vi "test motor reactions.vi"(6 "testing?":bool, 8 "REF INPUT":cluster{T30[], T36[], T39[], T40[], T41[]}={[{"Device"=enum."USB 0"}], [{"DevStatus"={"status"=FALSE, "code"=0, "source"=""}, "EncoderIndex"=enum."Enc 0", "CounterIndex"=enum."Invalid", "DistancePerCount"=0.026179938779914938, "Decoding Type"=enum."4x"}, {"DevStatus"={"status"=FALSE, "code"=0, "source"=""}, "EncoderIndex"=enum."Enc 1", "CounterIndex"=enum."Invalid", "DistancePerCount"=0.026179938779914938, "Decoding Type"=enum."4x"}], [], [], []}, 9 "REF OUTPUT":cluster{T32[], T42[], T43[]}, 10 "HARDWARE cluster":T1={"DRIVE MOTORS"=[], "Controller"=[], "ENCODERS"=[], "GYRO HARDWARE"={"Descr"="GYRO", "Installed?"=FALSE, "SPI Bus"=enum."SPI On-Board, CS0", "AnalogChannel"=enum."AI 0", "Calibrate On Open"=TRUE, "Calibrated Center Voltage"=0.0, "Calibration Time (s)"=2.0, "Sample Rate (Hz)"=100.0, "RefName"="", "stack name"="GYRO"}, "AIR"={"PRESSURE"=[], "COMPRESSOR"={"Descr"="COMPRESSOR", "Installed?"=TRUE, "Pneumatics Control Module"=0, "RefName"="COMPRESSOR", "stack name"="COMPRESSOR"}, "SOLENOIDS"=[]}, "MOTORS"=[], "SERVOS"=[], "SONAR"=[], "RELAY"=[], "LIMIT"=[]} {"MOTORS"."CAN ID" min=1 max=62 step=1; "MOTORS"."Motor Controller" items=["SPARK MAX", "SPARK", "Existing", "SD540", "TALON SRX", "VICTOR SP", "TALON SR", "JAGUAR", "VICTOR"]; "AIR"."PRESSURE"."warning HIGH" format="%.2f"; "AIR"."PRESSURE"."warning LOW" format="%.2f"; "AIR"."PRESSURE"."nominal value" format="%.2f"; "DRIVE MOTORS"."CAN ID" min=1 max=62 step=1; "DRIVE MOTORS"."Motor Controller" items=["SPARK MAX", "SPARK", "Existing", "SD540", "TALON SRX", "VICTOR SP", "TALON SR", "JAGUAR", "VICTOR"]; "Controller"."Parameters"."DEADBAND" format="%#_13g"; "Controller"."Parameters"."MIN SPEED" format="%#_13g"; "Controller"."Parameters"."MAX LIMIT" format="%#_13g"}, 11 "REF DRIVE JOYSTICK":T35={"JoystickDevRef"={"Device"=enum."USB 0"}, "RobotDriveDevRef"={"DevStatus"={"status"=FALSE, "code"=0, "source"=""}, "Motors[]"=[{"DeviceStatus"={"status"=FALSE, "code"=0, "source"=""}, "Type"=enum."PWM", "PWM"={"PWM Channel"=enum."PWM 0", "DeadBand"={"Name"="Victor SP", "maxPositivePwm"=230, "minPositivePwm"=154, "centerPwm"=153, "maxNegativePwm"=152, "minNegativePwm"=76, "angularRange"=0}}, "CAN"={"Device Number"=0, "SetOutput VI Ref"=variant(enum8{"Percent VBus", "Current", "Speed", "Position", "Voltage"} enum."Percent VBus"), "GetOutput VI Ref"=variant(refnum<k1> refnum), "Enable VI Ref"=variant(dbl 0.0), "Disable VI Ref"=variant(enum8{"Percent VBus", "Speed", "Position", "Slave", "Unchanged / Invalid"} enum."Percent VBus"), "Data"=variant}, "Invert"=FALSE, "DIO PWM"={"PWM \"Enable\" Channel"=enum."Invalid", "DIOChannel"=enum."Invalid", "PWM Rate"=0.0}}, {"DeviceStatus"={"status"=FALSE, "code"=0, "source"=""}, "Type"=enum."PWM", "PWM"={"PWM Channel"=enum."PWM 1", "DeadBand"={"Name"="Victor SP", "maxPositivePwm"=230, "minPositivePwm"=154, "centerPwm"=153, "maxNegativePwm"=152, "minNegativePwm"=76, "angularRange"=0}}, "CAN"={"Device Number"=0, "SetOutput VI Ref"=variant(enum8{"Percent VBus", "Current", "Speed", "Position", "Voltage"} enum."Percent VBus"), "GetOutput VI Ref"=variant(refnum<k1> refnum), "Enable VI Ref"=variant(dbl 0.0), "Disable VI Ref"=variant(enum8{"Percent VBus", "Speed", "Position", "Slave", "Unchanged / Invalid"} enum."Percent VBus"), "Data"=variant}, "Invert"=TRUE, "DIO PWM"={"PWM \"Enable\" Channel"=enum."Invalid", "DIOChannel"=enum."Invalid", "PWM Rate"=0.0}}], "Square Inputs"=TRUE, "Max Output"=1.0}}) -> (2 "Cluster":cluster{"LEFT":dbl, "RIGHT":dbl}={"LEFT"=155.04062951459707, "RIGHT"=154.7082225850084})   [LabVIEW 2019]
uses:
  <vilib>/Rock Robotics/WPI/MotorControl/WPI_MotorControlDeviceRef.ctl
  <vilib>/Rock Robotics/WPI/MotorControl/WPI_MotorControlType.ctl
  <vilib>/Rock Robotics/SystemInterfaces/DIO/FPGA_DIOPWMChannel.ctl
  <vilib>/Rock Robotics/WPI/PWM/WPI_PWMDeadband.ctl
  <vilib>/Rock Robotics/SystemInterfaces/DIO/FPGA_DIOChannel.ctl
  <vilib>/Rock Robotics/WPI/PWM/Servo/WPI_ServoDeviceRef.ctl
  <vilib>/Rock Robotics/WPI/Relay/WPI_RelayDevRef.ctl
  <vilib>/Rock Robotics/SystemInterfaces/DIO/FPGA_DIORelayChannel.ctl
  <vilib>/Rock Robotics/WPI/Relay/WPI_RelayDirection.ctl
  <vilib>/Rock Robotics/WPI/Joystick/WPI_JoystickDevRef.ctl
  <vilib>/Rock Robotics/WPI/Joystick/WPI_JoystickDeviceEnum.ctl
  <vilib>/Rock Robotics/WPI/Encoder/WPI_EncoderDevRef.ctl
  <vilib>/Rock Robotics/SystemInterfaces/Encoder/FPGA_EncoderIdx.ctl
  <vilib>/Rock Robotics/SystemInterfaces/Counter/FPGA_CounterCtrSystemIndex.ctl
  <vilib>/Rock Robotics/WPI/Encoder/WPI_EncoderType.ctl
  <vilib>/Rock Robotics/WPI/Ultrasonic/WPI_UltrasonicDeviceRef.ctl
  <vilib>/Rock Robotics/WPI/Switch/WPI_SwitchDevRef.ctl
  <vilib>/Rock Robotics/WPI/AnalogChannel/WPI_AnalogChannelDevRef.ctl
  <vilib>/Rock Robotics/SystemInterfaces/AI/FPGA_AIChannel.ctl
  <vilib>/Rock Robotics/WPI/RobotDrive/WPI_RobotDriveDevRef.ctl
  Controls/def HARDWARE CTRL info.ctl
  Controls/def MOTOR info.ctl
  Controls/ctrl MOTOR CTRLR SELECT.ctl
  <vilib>/Rock Robotics/WPI/ThirdParty/REV Robotics/SPARK MAX/Typedef/Spark MAX Motor Type.ctl
  Controls/def USER CONTROL info.ctl
  Controls/def JOYSTICK PARAMETERS.ctl
  Controls/def ENCODER info.ctl
  Controls/def GYRO info.ctl
  <vilib>/Rock Robotics/SystemInterfaces/spilib/spi_bus.ctl
  Controls/ctrl ANALOG CHANNEL SELECT.ctl
  Controls/def AIR PRESSURE info.ctl
  Controls/def COMPRESSOR info.ctl
  Controls/def SOLENOID info.ctl
  <vilib>/Rock Robotics/WPI/Solenoid/WPI_SolenoidChannel.ctl
  <vilib>/Rock Robotics/WPI/Solenoid/WPI_SolenoidValue.ctl
  Controls/def SERVO info.ctl
  Controls/def SONAR info.ctl
  Controls/ctrl SONAR DEVICE SELECT.ctl
  <vilib>/Rock Robotics/WPI/Ultrasonic/WPI_UltrasonicRangeUnits.ctl
  Controls/def RELAY info.ctl
  <vilib>/Rock Robotics/WPI/Relay/WPI_RelayValue.ctl
  Controls/def LIMIT SWITCH info.ctl
  Controls/ctrl ENCODER SELECT.ctl
panel:
  in  "milliseconds to wait":u32=25
  in  "INNER LOOPS":i32=50
  out "v":cluster{"LEFT":dbl, "RIGHT":dbl}={"LEFT"=34.73439216613769, "RIGHT"=34.65523719787597}
  out "x":cluster{"LEFT":dbl, "RIGHT":dbl}={"LEFT"=155.04062951459707, "RIGHT"=154.7082225850084}
  out "size(s)":i32=2
  out "Waveform Chart":T44(graph)=[{11.395975494291633, "Numeric"=1.0, "LEFT"=155.04062951459707, "RIGHT"=154.7082225850084, "LEFT"=34.73439216613769, "RIGHT"=34.65523719787597}]
  out "elapsed t (s)":dbl=11.395975494291633 format="%.4f"
  out "delta t (s)":dbl=0.05002135713584721 format="%.4f"
  out "MOTOR VALUE":dbl=1.0
  out "motor profile":dbl[](array[numeric])=[0.0, 0.05, 0.1, 0.15000000000000002, 0.2, 0.25, 0.30000000000000004, 0.35000000000000003, 0.4, 0.45, 0.5, 0.55, 0.6000000000000001, 0.65, 0.7000000000000001, 0.75, 0.8, 0.8500000000000001, 0.9, 0.9500000000000001, 1.0] format="%.3f"
  in  "motor increment":dbl=0.05 format="%#_13g"
  in  "motor profile type":enum16{"unit pulse", "step"}(ring)
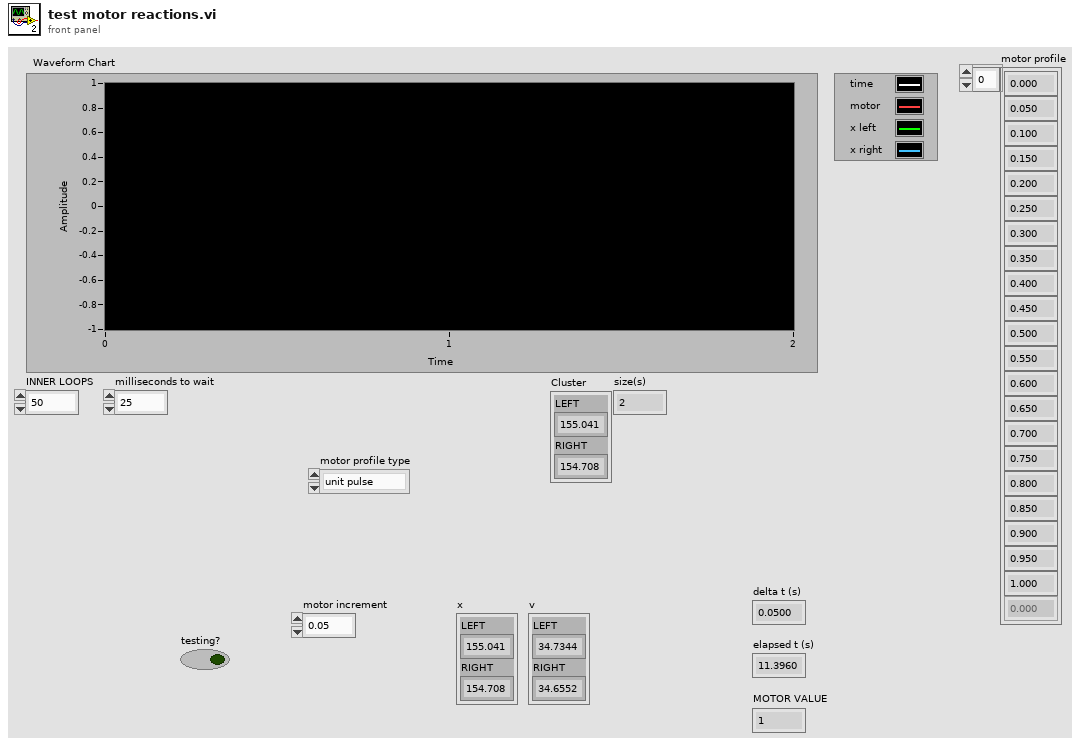
[diagram p1: front panel]
types:
  T1 = typedef "def HARDWARE CTRL info.ctl" = cluster{"DRIVE MOTORS":T2[], "Controller":T6[], "ENCODERS":T9[], "GYRO HARDWARE":T12, "AIR":cluster{"PRESSURE":T15[], "COMPRESSOR":T17, "SOLENOIDS":T18[]}, "MOTORS":T2[], "SERVOS":T21[], "SONAR":T22[], "RELAY":T25[], "LIMIT":T29[]}
  T2 = typedef "def MOTOR info.ctl" = cluster{"Descr":string, "Motor Controller":T3, "PWM ch":T4, "Invert?":bool, "Installed?":bool, "RefName":string, "stack name":string, "remove deadband":bool, "CAN ID":u8, "IDLE BEHAVIOUR":string, "Motor Type":T5}
  T3 = typedef "ctrl MOTOR CTRLR SELECT.ctl" = u16
  T4 = typedef "FPGA_DIOPWMChannel.ctl" = enum8{"PWM 0", "PWM 1", "PWM 2", "PWM 3", "PWM 4", "PWM 5", "PWM 6", "PWM 7", "PWM 8", "PWM 9", "PWM MXP 0", "PWM MXP 1", "PWM MXP 2", "PWM MXP 3", "PWM MXP 4", "PWM MXP 5", "PWM MXP 6", "PWM MXP 7", "PWM MXP 8", "PWM MXP 9", "Invalid"}
  T5 = typedef "Spark MAX Motor Type.ctl" = enum16{"Brushed", "Brushless"}
  T6 = typedef "def USER CONTROL info.ctl" = cluster{"Descr":string, "Installed?":bool, "RefName":string, "JoystickDevice":T7, "Invert Y axis":bool, "Scale":dbl, "AXIS":string, "BUTTONS":string, "POV":string, "Parameters":T8}
  T7 = typedef "WPI_JoystickDeviceEnum.ctl" = enum16{"USB 0", "USB 1", "USB 2", "USB 3", "USB 4", "USB 5"}
  T8 = typedef "def JOYSTICK PARAMETERS.ctl" = cluster{"MAX LIMIT":dbl, "MIN SPEED":dbl, "DEADBAND":dbl, "invert X?":bool, "invert Y?":bool}
  T9 = typedef "def ENCODER info.ctl" = cluster{"Descr":string, "Installed?":bool, "A Channel":T10, "B Channel":T10, "Invert Direction":bool, "Enum":T11, "Gear ratio":dbl, "Cycles per Rev":dbl, "Diameter (in)":dbl[unit], "RefName":string, "stack name":string, "min rate (hz)":dbl, "Samples":u8, "STACK subnames":cluster{"RESET name":string, "STOPPED name":string, "DIRECTION name":string, "RATE name":string, "INSTALLED name":string}}
  T10 = typedef "FPGA_DIOChannel.ctl" = enum8{"DIO 0", "DIO 1", "DIO 2", "DIO 3", "DIO 4", "DIO 5", "DIO 6", "DIO 7", "DIO 8", "DIO 9", "DIO MXP 0", "DIO MXP 1", "DIO MXP 2", "DIO MXP 3", "DIO MXP 4", "DIO MXP 5", "DIO MXP 6", "DIO MXP 7", "DIO MXP 8", "DIO MXP 9", "DIO MXP 10", "DIO MXP 11", "DIO MXP 12", "DIO MXP 13", "DIO MXP 14", "DIO MXP 15", "SPI Port CS1", "SPI Port CS2", "SPI Port CS3", "SPI Port MISO", "SPI Port MOSI", "Invalid"}
  T11 = typedef "WPI_EncoderType.ctl" = enum16{"1x", "2x", "4x"}
  T12 = typedef "def GYRO info.ctl" = cluster{"Descr":string, "Installed?":bool, "SPI Bus":T13, "AnalogChannel":T14, "Calibrate On Open":bool, "Calibrated Center Voltage":dbl, "Calibration Time (s)":dbl, "Sample Rate (Hz)":dbl, "RefName":string, "stack name":string}
  T13 = typedef "spi_bus.ctl" = enum16{"SPI On-Board, CS0", "SPI On-Board, CS1", "SPI On-Board, CS2", "SPI On-Board, CS3", "SPI MXP", "Invalid"}
  T14 = typedef "ctrl ANALOG CHANNEL SELECT.ctl" = enum8{"AI 0", "AI 1", "Invalid"}
  T15 = typedef "def AIR PRESSURE info.ctl" = cluster{"Descr":string, "Installed?":bool, "Channel":T16, "RefName":string, "stack name":string, "MULTIPLIER":dbl, "OFFSET":dbl, "nominal value":dbl, "warning LOW":dbl, "warning HIGH":dbl}
  T16 = typedef "FPGA_AIChannel.ctl" = enum8{"AI 0", "AI 1", "AI 2", "AI 3", "AI MXP 0", "AI MXP 1", "AI MXP 2", "AI MXP 3", "Invalid"}
  T17 = typedef "def COMPRESSOR info.ctl" = cluster{"Descr":string, "Installed?":bool, "Pneumatics Control Module":u8, "RefName":string, "stack name":string}
  T18 = typedef "def SOLENOID info.ctl" = cluster{"Descr":string, "Installed?":bool, "Pneumatics Control Module (0)":u8, "DBL":bool, "SolenoidChannel":T19, "SolenoidChannel":T19, "Default SET":T20, "RefName":string, "Value":string}
  T19 = typedef "WPI_SolenoidChannel.ctl" = enum8{"Solenoid 0", "Solenoid 1", "Solenoid 2", "Solenoid 3", "Solenoid 4", "Solenoid 5", "Solenoid 6", "Solenoid 7", "Invalid"}
  T20 = typedef "WPI_SolenoidValue.ctl" = enum16{"Off", "On", "Forward", "Reverse"}
  T21 = typedef "def SERVO info.ctl" = cluster{"Descr":string, "PWM ch":T4, "Installed?":bool, "Angular range":dbl, "RefName":string, "stack name":string}
  T22 = typedef "def SONAR info.ctl" = cluster{"Descr":string, "Installed?":bool, "Device type":T23, "PING Channel":T10, "ECHO Channel":T10, "RefName":string, "stack name":string, "Samples":i32, "Range Units":T24}
  T23 = typedef "ctrl SONAR DEVICE SELECT.ctl" = enum16{"SRF04 Digital", "MB1010 Digital", "MB1010 Analog", "SRF08 Digital"}
  T24 = typedef "WPI_UltrasonicRangeUnits.ctl" = enum16{"inches", "mm"}
  T25 = typedef "def RELAY info.ctl" = cluster{"Descr":string, "Installed?":bool, "RelayChannel":T26, "Relay Direction":T27, "Relay Value":T28, "RefName":string, "Value":string}
  T26 = typedef "FPGA_DIORelayChannel.ctl" = enum8{"Relay 0", "Relay 1", "Relay 2", "Relay 3", "Invalid"}
  T27 = typedef "WPI_RelayDirection.ctl" = enum16{"Both directions", "Forward only", "Reverse only"}
  T28 = typedef "WPI_RelayValue.ctl" = enum16{"Off", "On", "Forward", "Reverse"}
  T29 = typedef "def LIMIT SWITCH info.ctl" = cluster{"Descr":string, "Installed?":bool, "A Channel":T10, "Normally Closed?":bool, "RefName":string, "stack name":string}
  T30 = typedef "WPI_JoystickDevRef.ctl" = cluster{"Device":T7}
  T31 = typedef "WPI_RobotDriveDevRef.ctl" = cluster{"DevStatus":errorcluster, "Motors[]":T32[], "Square Inputs":bool, "Max Output":dbl}
  T32 = typedef "WPI_MotorControlDeviceRef.ctl" = cluster{"DeviceStatus":errorcluster, "Type":T33, "PWM":cluster{"PWM Channel":T4, "DeadBand":T34}, "CAN":cluster{"Device Number":u8, "SetOutput VI Ref":variant, "GetOutput VI Ref":variant, "Enable VI Ref":variant, "Disable VI Ref":variant, "Data":variant}, "Invert":bool, "DIO PWM":cluster{"PWM \"Enable\" Channel":T4, "DIOChannel":T10, "PWM Rate":dbl}}
  T33 = typedef "WPI_MotorControlType.ctl" = enum16{"PWM", "CAN", "DIO PWM"}
  T34 = typedef "WPI_PWMDeadband.ctl" = cluster{"Name":string, "maxPositivePwm":i32, "minPositivePwm":i32, "centerPwm":i32, "maxNegativePwm":i32, "minNegativePwm":i32, "angularRange":u16}
  T35 = cluster{"JoystickDevRef":T30, "RobotDriveDevRef":T31}
  T36 = typedef "WPI_EncoderDevRef.ctl" = cluster{"DevStatus":errorcluster, "EncoderIndex":T37, "CounterIndex":T38, "DistancePerCount":dbl, "Decoding Type":T11}
  T37 = typedef "FPGA_EncoderIdx.ctl" = enum8{"Enc 0", "Enc 1", "Enc 2", "Enc 3", "Enc 4", "Enc 5", "Enc 6", "Enc 7", "Invalid"}
  T38 = typedef "FPGA_CounterCtrSystemIndex.ctl" = enum8{"Ctr 0", "Ctr 1", "Ctr 2", "Ctr 3", "Ctr 4", "Ctr 5", "Ctr 6", "Ctr 7", "Invalid"}
  T39 = typedef "WPI_UltrasonicDeviceRef.ctl" = cluster{"DevStatus":errorcluster, "Ping Channel":T10, "Echo Channel":T10, "CntIndex":T38}
  T40 = typedef "WPI_SwitchDevRef.ctl" = cluster{"DevStatus":errorcluster, "DIO Channel":T10, "CntIndex":T38, "Normally Closed":bool}
  T41 = typedef "WPI_AnalogChannelDevRef.ctl" = cluster{"DevStatus":errorcluster, "Analog Channel":T16}
  T42 = typedef "WPI_ServoDeviceRef.ctl" = cluster{"DeviceStatus":errorcluster, "PWM Channel":T4, "DeadBand":T34}
  T43 = typedef "WPI_RelayDevRef.ctl" = cluster{"DevStatus":errorcluster, "Relay Channel":T26, "Relay Direction":T27}
  T44 = cluster{dbl, "Numeric":dbl, "LEFT":dbl, "RIGHT":dbl, "LEFT":dbl, "RIGHT":dbl}[]
  T45 = cluster{dbl, "Numeric":dbl, "LEFT":dbl, "RIGHT":dbl, "LEFT":dbl, "RIGHT":dbl}
  T46 = typedef "ctrl ENCODER SELECT.ctl" = u16
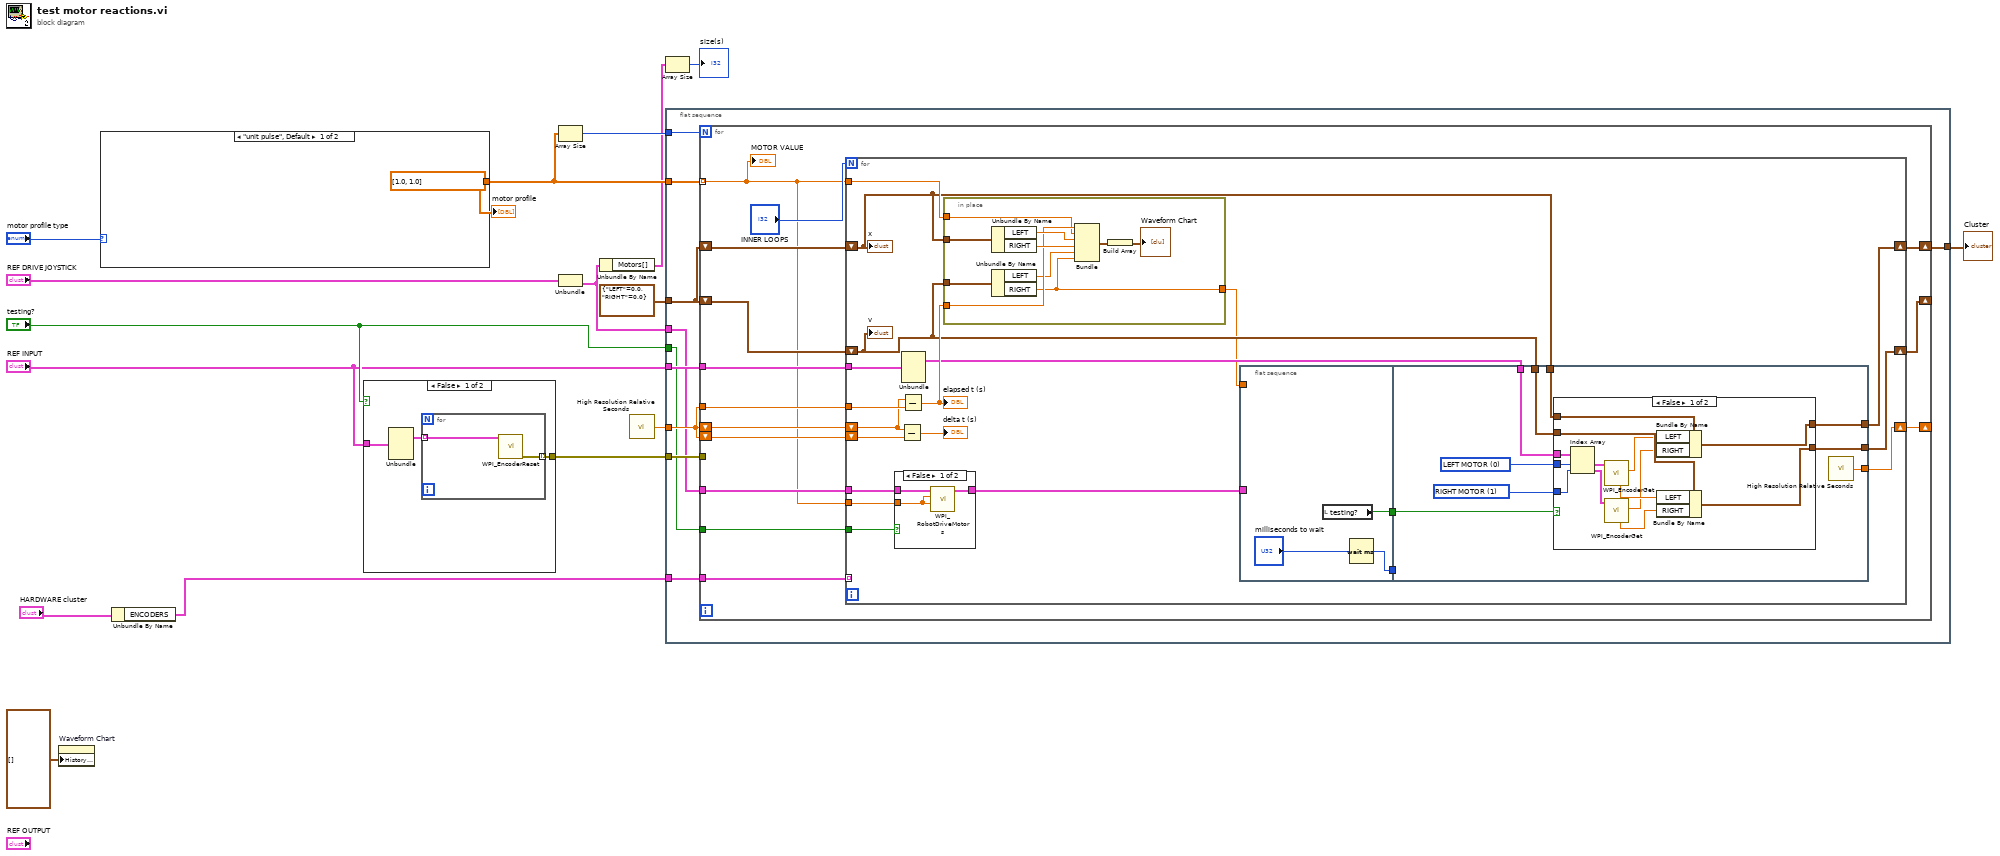
[diagram p0: block diagram]
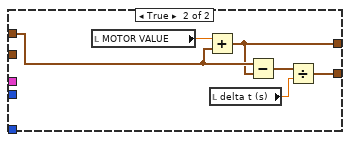
[diagram p4: hidden frame]
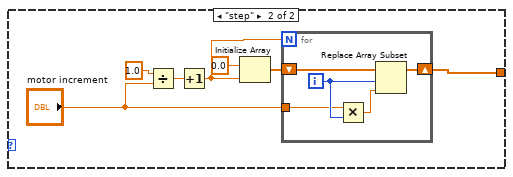
[diagram p5: hidden frame]
diagram:
  n1 = property on="Waveform Chart" class="WFChart (strict)"("History Data"=T44 []) -> ()  [unwired: 2 in, 2 out]
  n2 = case shown="\"unit pulse\", Default" "motor profile type" {
    tunnel: [dbl[] [1.0, 1.0] w22] -> w14
    frame "unit pulse", Default {
    }
    frame "step" {
      n3 = Divide(x=1.0, y="motor increment") -> (x/y=w23:dbl)
      n4 = Increment(x=w23) -> (x+1=w19:dbl)
      n5 = Initialize Array(0.0, w19) -> (w20:dbl[])
      n6 = for {
        N: w19 -> [_]
        shift-right: [w29] -> w22
        shift-left: w20 -> [w28]
        tunnel: "motor increment" -> [w25]
        i -> [w26]
        n7 = Multiply(x=w25, y=w26) -> (x*y=w27:dbl)
        n8 = Replace Array Subset(array=w28, new element=w27, index=w26) -> (w29:dbl[])
      }
    }
  }
  "motor profile" <- w14
  n9 = Unbundle By Name("HARDWARE cluster") -> ("ENCODERS"=w1:T9[])
  n10 = case shown="False" "testing?" {
    tunnel: "REF INPUT" -> [w32 _]
    tunnel: [w30 _] -> w4
    frame False {
      n11 = Unbundle(w32) -> (w31:T36[])  [unwired: 4 out]
      n12 = for {
        tunnel: w31 -> [w33] mode=indexing
        tunnel: [w34] -> w30 mode=indexing
        n13 = call <vilib>:"WPI_EncoderReset.vi"("EncoderDevRef"=w33) -> ("error out"=w34:errorcluster)  [unwired: 9 in, 1 out]
      }
    }
    frame True {
    }
  }
  n14 = Array Size(array=w14) -> (size(s)=w15:i32)
  n15 = Unbundle("REF DRIVE JOYSTICK") -> ("RobotDriveDevRef"=w9:T31)  [unwired: 1 out]
  n16 = Unbundle By Name(w9) -> ("Motors[]"=w8:T32[])
  n17 = call <vilib>:"High Resolution Relative Seconds.vi"() -> ("relative seconds"=w12:dbl)
  n18 = Array Size(array=w8) -> (size(s)=→"size(s)":i32)
  n19 = flat-sequence {
    tunnel: w15 -> [w44]
    tunnel: w14 -> [w43]
    tunnel: cluster{"LEFT":dbl, "RIGHT":dbl} {"LEFT"=0.0, "RIGHT"=0.0} -> [w38]
    tunnel: w12 -> [w40]
    tunnel: w9 -> [w36]
    tunnel: "testing?" -> [w37]
    tunnel: "REF INPUT" -> [w42]
    tunnel: [w41] -> w10
    tunnel: w4 -> [w39]
    tunnel: w1 -> [w35]
    frame #0 {
      n20 = for {
        N: w44 -> [_]
        tunnel: w43 -> [w46] mode=indexing
        shift-right: [w56] -> w41
        shift-left: w38 -> [w58]
        shift-right: [w57] -> _
        shift-left: w38 -> [w50]
        shift-right: [w54] -> _
        shift-left: w40 -> [w52]
        tunnel: w40 -> [w55]
        tunnel: w42 -> [w53]
        shift-left: w40 -> [w51]
        tunnel: w39 -> [_]
        tunnel: w37 -> [w48]
        tunnel: w36 -> [w47]
        tunnel: w35 -> [w45]
        n21 = for {
          N: "INNER LOOPS" -> [_]
          shift-right: [w64] -> w56
          shift-left: w58 -> [w65]
          shift-right: [w66] -> w57
          shift-left: w50 -> [w67]
          shift-right: [w68] -> w54
          shift-left: w52 -> [w77]
          tunnel: w55 -> [w78]
          shift-left: w51 -> [w76]
          tunnel: w46 -> [w73]
          tunnel: w53 -> [w71]
          tunnel: w48 -> [w62]
          tunnel: w47 -> [w61]
          tunnel: w46 -> [w60]
          tunnel: w45 -> [_] mode=indexing
          n22 = case shown="False" w62 {
            tunnel: w61 -> [w81 _]
            tunnel: w60 -> [w79 _]
            tunnel: [w80 _] -> w59
            frame False {
              n23 = call <vilib>:"WPI_RobotDriveMotors.vi"("RightSpeed"=w79, "LeftSpeed"=w79, "RobotDriveDevRef"=w81) -> ("RobotDriveDevRef"=w80:T31)  [unwired: 6 in, 2 out]
            }
            frame True {
            }
          }
          n24 = Subtract(x=w77, y=w76) -> (x-y=→"delta t (s)":dbl)
          n25 = Subtract(x=w77, y=w78) -> (x-y=w74:dbl)
          "elapsed t (s)" <- w74
          n26 = Unbundle(w71) -> (w70:T36[])  [unwired: 4 out]
          n27 = in-place {
            in-place-border: w65 -> [w89]
            in-place-border: w74 -> [w86]
            in-place-border: w73 -> [w85]
            in-place-border: w67 -> [w83]
            in-place-border: [w82] -> w63
            n28 = Unbundle By Name(w89) -> ("LEFT"=w88:dbl, "RIGHT"=w87:dbl)
            n29 = Unbundle By Name(w83) -> ("LEFT"=w84:dbl, "RIGHT"=w82:dbl)
            n30 = Bundle(w86, "Numeric"=w85, "LEFT"=w88, "RIGHT"=w87, "LEFT"=w84, "RIGHT"=w82) -> (w90:T45)  [unwired: 1 in]
            n31 = Build Array(w90) -> (→"Waveform Chart":T44)
          }
          n32 = flat-sequence {
            tunnel: [w93] -> w72
            tunnel: [w92] -> w69
            tunnel: w63 -> [_]
            tunnel: w59 -> [_]
            tunnel: w72 -> [_]
            tunnel: w70 -> [w102]
            tunnel: w69 -> [w103]
            tunnel: w67 -> [w99]
            tunnel: [w98] -> w68
            tunnel: [w97] -> w66
            tunnel: w65 -> [w96]
            tunnel: [w95] -> w64
            frame #0 {
              n33 = local read "testing?"() -> (w92:bool)
              n34 = Wait (ms)(milliseconds to wait="milliseconds to wait") -> (millisecond timer value=w93:u32)
            }
            frame #1 {
              w100 = T46 1 items=["LEFT MOTOR", "RIGHT MOTOR"] ("SELECT ENCODER")
              w101 = T46 0 items=["LEFT MOTOR", "RIGHT MOTOR"] ("SELECT ENCODER")
              n35 = case shown="False" w103 {
                tunnel: w102 -> [w114 _]
                tunnel: w101 -> [w116 _]
                tunnel: w100 -> [w115 _]
                tunnel: w99 -> [w111 _]
                tunnel: [w110 w117] -> w97
                tunnel: w96 -> [w106 w120]
                tunnel: [w107 w119] -> w95
                frame False {
                  n36 = Index Array(array=w114, index #1=w116, index #2=w115) -> (element #1=w113:T36, element #2=w112:T36)
                  n37 = call <vilib>:"WPI_EncoderGet.vi"("EncoderDevRef"=w113) -> ("Distance"=w105:dbl, "Rate"=w109:dbl)  [unwired: 5 in, 4 out]
                  n38 = call <vilib>:"WPI_EncoderGet.vi"("EncoderDevRef"=w112) -> ("Distance"=w104:dbl, "Rate"=w108:dbl)  [unwired: 5 in, 4 out]
                  n39 = Bundle By Name(cluster=w106, "LEFT"=w105, "RIGHT"=w104) -> (w107:cluster{"LEFT":dbl, "RIGHT":dbl})
                  n40 = Bundle By Name(cluster=w111, "LEFT"=w109, "RIGHT"=w108) -> (w110:cluster{"LEFT":dbl, "RIGHT":dbl})
                }
                frame True {
                  n41 = local read "MOTOR VALUE"() -> (w122:dbl)
                  n42 = Add(x=w122, y=w120) -> (x+y=w119:cluster{"LEFT":dbl, "RIGHT":dbl})
                  n43 = local read "delta t (s)"() -> (w121:dbl)
                  n44 = Subtract(x=w120, y=w119) -> (x-y=w118:cluster{"LEFT":dbl, "RIGHT":dbl})
                  n45 = Divide(x=w118, y=w121) -> (x/y=w117:cluster{"LEFT":dbl, "RIGHT":dbl})
                }
              }
              n46 = call <vilib>:"High Resolution Relative Seconds.vi"() -> ("relative seconds"=w98:dbl)
            }
          }
          "x" <- w65
          "v" <- w67
        }
        "MOTOR VALUE" <- w46
      }
    }
  }
  "Cluster" <- w10
